vi "Launcher Preperation.vi"() -> (1 "READY!":bool)   [LabVIEW 2012]
uses:
  BotStatus.vi
  Motors Values.vi
  <vilib>/express/express arith-compare/Formula/XNode/ExpressFormulaBlockNode.xnode
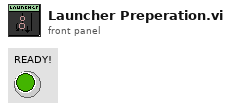
[diagram p1: front panel]
types:
  T1 = cluster{"Middle":bool, "Cannon":bool, "InFlipper":bool, "FlipperAtPlace":bool, "Bottom":bool, "FrisbeeDirection":bool}
  T2 = typedef "WPI_EncoderDevRef.ctl" = cluster{"DevStatus":errorcluster, "EncoderIndex":T3, "CounterIndex":T4, "DistancePerCount":dbl, "Decoding Type":T5}
  T3 = typedef "FPGA_EncoderIdx.ctl" = enum8{"Enc 0", "Enc 1", "Enc 2", "Enc 3", "Invalid"}
  T4 = typedef "FPGA_CounterCtrSystemIndex.ctl" = enum8{"Ctr 0", "Ctr 1", "Ctr 2", "Ctr 3", "Ctr 4", "Ctr 5", "Ctr 6", "Ctr 7", "Invalid"}
  T5 = typedef "WPI_EncoderType.ctl" = enum16{"1x", "2x", "4x"}
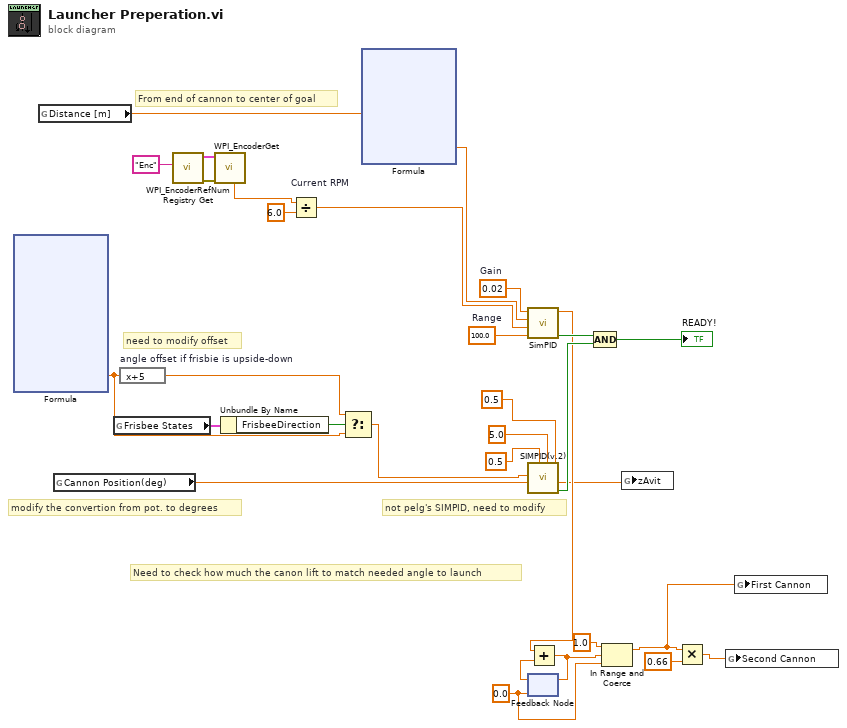
[diagram p0: block diagram]
diagram:
  w11 = 0.0
  w19 = 100.0  # Range
  w20 = 0.02  # Gain
  # "From end of cannon to center of goal"
  # "need to modify offset"
  # "not pelg's SIMPID, need to modify"
  # "modify the convertion from pot. to degrees"
  # "Need to check how much the canon lift to match needed angle to launch"
  n1 = xnode "Formula"() -> ("Result"=w9:dbl)  [unwired: 5 in, 1 out]
  n2 = global read "BotStatus.vi" "Distance [m]"() -> (w6:dbl)
  n3 = global read "BotStatus.vi" "Cannon Position(deg)"() -> (w7:dbl)
  n4 = global read "BotStatus.vi" "Frisbee States"() -> (w5:T1)
  n5 = expression code="x+5" "angle offset if frisbie is upside-down"(w9) -> (w8:dbl)
  n6 = call <vilib>:"WPI_EncoderRefNum Registry Get.vi"("refnum name"="Enc") -> ("error out"=w24:errorcluster, "EncoderDevRef"=w25:T2)  [unwired: 9 in]
  n7 = call <vilib>:"WPI_EncoderGet.vi"("error in (no error)"=w24, "EncoderDevRef"=w25) -> ("Rate"=w22:dbl)  [unwired: 4 in, 5 out]
  n8 = Unbundle By Name(w5) -> ("FrisbeeDirection"=w4:bool)
  n9 = Divide "Current RPM"(x=w22, y=6.0) -> (x/y=w18:dbl)
  n10 = Select(t=w8, s=w4, f=w9) -> (s? t:f=w10:dbl)
  n11 = xnode "Formula"("D"=w6) -> ("Result"=w17:dbl)  [unwired: 2 in, 1 out]
  n12 = call "SimPID.vi"("Range"=w19, "Position"=w18, "Set Point"=w17, "Gain"=w20) -> ("On Target"=w16:bool, "result"=w15:dbl)  [unwired: 5 in]
  n13 = call "SIMPID(v.2).vi"("Range"=0.5, "upper limit"=5.0, "lower limit"=0.5, "Current Point"=w7, "Set Point"=w10) -> ("On Target"=w29:bool, "result"=w1:dbl)  [unwired: 5 in]
  n14 = feedback #1(w11) -> (w14:dbl)
  n15 = Add(x=w15, y=w14) -> (x+y=w13:dbl)
  n16 = feedback-in #1(w13) -> ()
  n17 = Compound Arithmetic op=AND(w16, w29) -> (→"READY!":bool)
  n18 = In Range and Coerce(upper limit=1.0, x=w13, lower limit=w11) -> (coerced(x)=w2:dbl)  [unwired: 1 out]
  n19 = global write "Motors Values.vi" "zAvit"(w1) -> ()
  n20 = Multiply(x=w2, y=0.66) -> (x*y=w3:dbl)
  n21 = global write "Motors Values.vi" "Second Cannon"(w3) -> ()
  n22 = global write "Motors Values.vi" "First Cannon"(w2) -> ()
